vi "FunctDataMgr.Read Mode.vi"(8 "error in (no error)":errorcluster, 11 "FunctDataMgr in":refnum<class "FunctDataMgr.lvclass">) -> (0 "error out":errorcluster, 1 "SN":string, 2 "Sequence":string, 3 "FunctDataMgr out":refnum<class "FunctDataMgr.lvclass">, 4 "StartTime":timestamp, 5 "Mode":string, 6 "Pos":i32)   [LabVIEW 2024, in "FunctDataMgr.lvclass"]
uses:
  FunctDataMgr.lvclass
  FunctDataMgr.lvclass/FunctDataMgr.ctl
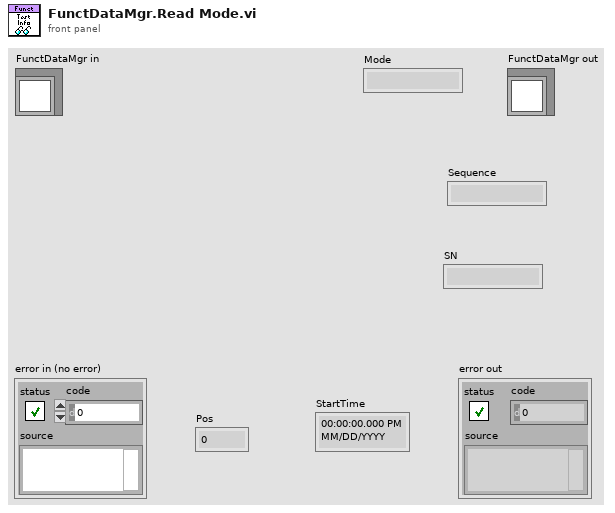
[diagram p1: front panel]
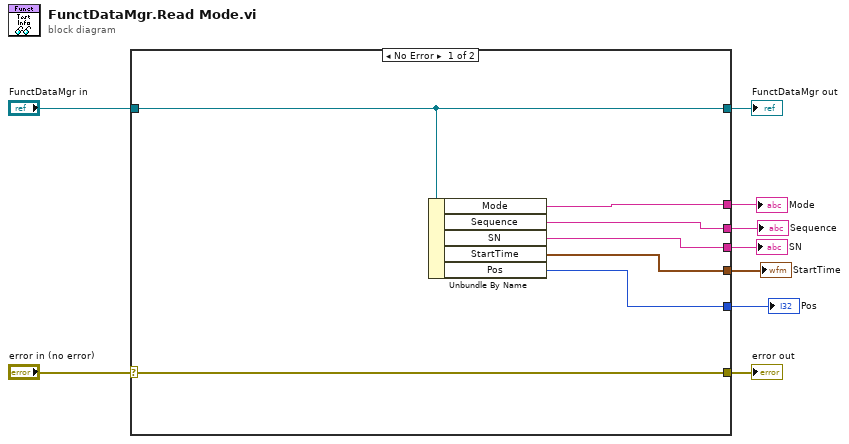
[diagram p0: block diagram]
diagram:
  n1 = case shown="No Error" "error in (no error)" {
    selector: "error in (no error)" -> [w16 w18]
    tunnel: [w16 w18] -> w8
    tunnel: [w15 w17] -> w6
    tunnel: "FunctDataMgr in" -> [w15 w17]
    tunnel: [w14 _] -> w5
    tunnel: [w13 _] -> w4
    tunnel: [w12 _] -> w3
    tunnel: [w11 _] -> w2
    tunnel: [w10 _] -> w1
    frame No Error {
      n2 = Unbundle By Name(w15) -> ("Mode"=w14:string, "Sequence"=w12:string, "SN"=w11:string, "StartTime"=w13:timestamp, "Pos"=w10:i32)
    }
    frame Error {
    }
  }
  "error out" <- w8
  "FunctDataMgr out" <- w6
  "Mode" <- w5
  "Sequence" <- w3
  "SN" <- w2
  "StartTime" <- w4
  "Pos" <- w1
